vi "MouseEvents.vi"(11 "Mouse Event":T1=2 items=["MOUSEEVENTF_ABSOLUTE"=32768, "MOUSEEVENTF_LEFTDOWN"=2, "MOUSEEVENTF_LEFTUP"=4, "MOUSEEVENTF_MIDDLEDOWN"=32, "MOUSEEVENTF_MIDDLEUP"=64, "MOUSEEVENTF_MOVE"=1, "MOUSEEVENTF_RIGHTDOWN"=8, "MOUSEEVENTF_RIGHTUP"=16, "MOUSEEVENTF_WHEEL"=2048, "MOUSEEVENTF_XDOWN"=128, "MOUSEEVENTF_XUP"=256]) -> ()   [LabVIEW 2010]
uses:
  Mouse Events.ctl
  user32.dll
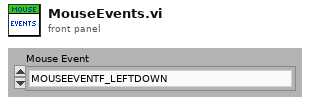
[diagram p1: front panel]
types:
  T1 = typedef "Mouse Events.ctl" = u32
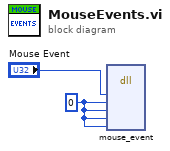
[diagram p0: block diagram]
diagram:
  w2 = u32 0 ("x")
  n1 = dll-call lib="user32.dll" fn="mouse_event"("flags"="Mouse Event", "x"=w2, "y"=w2, "data"=w2, "extraInfo"=w2) -> ()  [unwired: 9 in, 2 out]
